vi "AppendArray_9215.vi"(2 "Array Max Size":i32, 3 "Append Element":dbl, 4 "1D Array In":dbl[](array[numeric]), 5 "2D AppendArr":dbl[][](array[numeric]), 6 "2D ArrayIn":dbl[][](array[numeric])) -> (0 "1D Array Out":dbl[](array[numeric]), 1 "2D ArrayOut":dbl[][](array[numeric]))   [LabVIEW 2018]
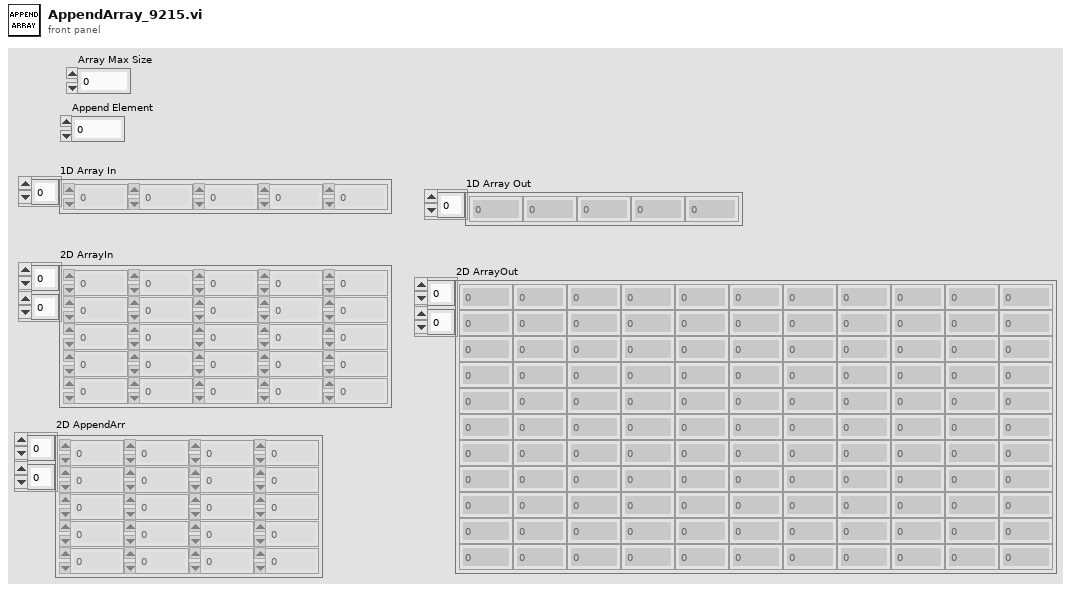
[diagram p1: front panel]
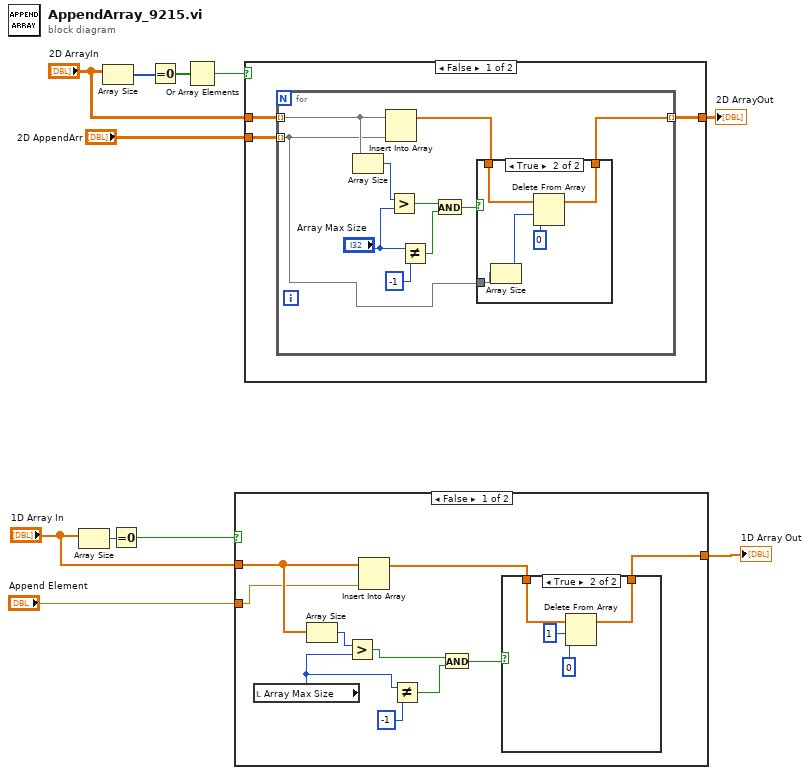
[diagram p0: block diagram]
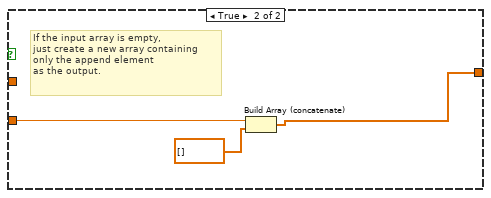
[diagram p3: hidden frame]
diagram:
  n1 = Array Size(array="1D Array In") -> (size(s)=w5:i32)
  n2 = Array Size(array="2D ArrayIn") -> (size(s)=w11:i32[])
  n3 = Equal To 0?(x=w5) -> (x = 0?=w4:bool)
  n4 = Equal To 0?(x=w11) -> (x = 0?=w10:bool[])
  n5 = Or Array Elements(Boolean array=w10) -> (logical OR=w9:bool)
  n6 = case shown="False" w4 {
    tunnel: "Append Element" -> [w14 w28]
    tunnel: [w12 w27] -> w2
    tunnel: "1D Array In" -> [w15 _]
    frame False {
      n7 = local read "Array Max Size"() -> (w19:i32)
      n8 = Array Size(array=w15) -> (size(s)=w21:i32)
      n9 = Greater?(x=w21, y=w19) -> (0:w17:bool)
      n10 = Insert Into Array(array=w15, new element=w14) -> (w13:dbl[])  [unwired: 1 in]
      n11 = Not Equal?(x=w19, y=-1) -> (x != y?=w18:bool)
      n12 = And(x=w17, y=w18) -> (x .and. y?=w16:bool)
      n13 = case shown="True" w16 {
        tunnel: w13 -> [w22 w26]
        tunnel: [w22 w25] -> w12
        frame False {
        }
        frame True {
          n14 = Delete From Array(array=w26, length=1, index=0) -> (array with subset deleted=w25:dbl[])  [unwired: 1 out]
        }
      }
    }
    frame True {
      # "If the input array is empty,\njust create a new array containing\nonly the append element\nas the output."
      n15 = Build Array (concatenate)(w28, dbl[] []) -> (w27:dbl[])
    }
  }
  "1D Array Out" <- w2
  n16 = case shown="False" w9 {
    tunnel: "2D ArrayIn" -> [w32 _]
    tunnel: "2D AppendArr" -> [w31 w49]
    tunnel: [w30 w49] -> w6
    frame False {
      n17 = for {
        tunnel: w32 -> [w41] mode=indexing
        tunnel: w31 -> [w37] mode=indexing
        tunnel: [w39] -> w30 mode=indexing
        n18 = Array Size(array=w41) -> (size(s)=w40:i32)
        n19 = Insert Into Array(array=w41, new element=w37) -> (w42:dbl[])  [unwired: 1 in]
        n20 = Greater?(x=w40, y="Array Max Size") -> (0:w35:bool)
        n21 = Not Equal?(x="Array Max Size", y=-1) -> (x != y?=w36:bool)
        n22 = And(x=w35, y=w36) -> (x .and. y?=w34:bool)
        n23 = case shown="True" w34 {
          tunnel: w37 -> [_ w48]
          tunnel: w42 -> [w43 w47]
          tunnel: [w43 w44] -> w39
          frame False {
          }
          frame True {
            n24 = Array Size(array=w48) -> (size(s)=w46:i32)
            n25 = Delete From Array(array=w47, length=w46, index=0) -> (array with subset deleted=w44:dbl[])  [unwired: 1 out]
          }
        }
      }
    }
    frame True {
      # "If the input array is empty,\njust use the append array\nas the output."
    }
  }
  "2D ArrayOut" <- w6
